vi "Write - Warning Input - Returns Same Warning.vi"() -> ()   [LabVIEW 2017, in "Generic Object Serializer Tests.lvlib" / "Serialization Binder.lvlib"]
uses:
  Serialization Binder.lvlib
  Generic Object Serializer/Generic Object Serializer.lvclass
  Serialization Binder/Serialization Binder.lvclass
  Generic Object Serializer/Write Serialization Binder.vi
  <vilib>/Utility/error.llb/Error Cluster From Error Code.vi
  <vilib>/ErrorRing/Error Ring.xnode
  <vilib>/addons/_JKI Toolkits/Caraya/classes/Test/Test.lvclass
  <vilib>/addons/_JKI Toolkits/Caraya/classes/Assert/Assert.lvclass
panel:
  out "error out":errorcluster
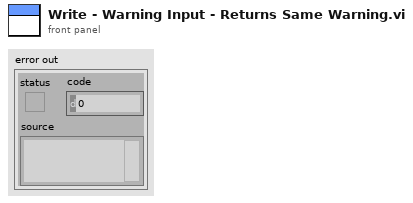
[diagram p1: front panel]
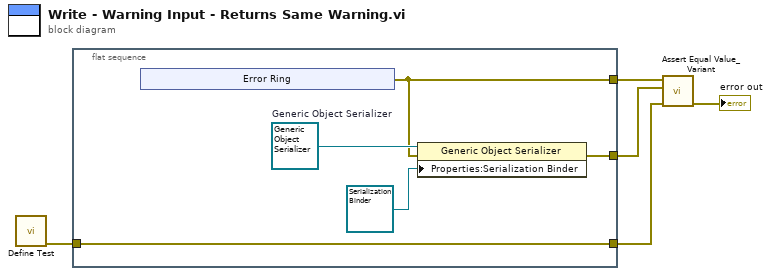
[diagram p0: block diagram]
diagram:
  n1 = call <vilib>:"Define Test.vi"() -> ("error out"=w4:errorcluster)  [unwired: 11 in]
  n2 = flat-sequence {
    tunnel: [w8] -> w5
    tunnel: w4 -> [w9]
    tunnel: [w9] -> w3
    tunnel: [w7] -> w1
    frame #0 {
      w10 = refnum<class "Generic Object Serializer.lvclass"> refnum  # Generic Object Serializer
      n3 = xnode "Error Ring"() -> ("error out"=w7:errorcluster)
      n4 = property class="Generic Object Serializer"(reference=w10, error in=w7, "Properties:Serialization Binder"=refnum<class "Serialization Binder.lvclass"> refnum ("Serialization Binder")) -> (error out=w8:errorcluster)  [unwired: 1 out]
    }
  }
  n5 = call <vilib>:"Assert Equal Value_Variant.vi"("error in (no error)"=w3, "Y"=w5, "X"=w1) -> ("error out"=→"error out":errorcluster)  [unwired: 8 in]
